vi "ShutdownCameraAndNIUSB.vi"(11 "Cluster":T3) -> ()   [LabVIEW 2024]
uses:
  <vilib>/vision/driver/NI_Vision_Acquisition_Software.lvlib
  <vilib>/userDefined/High Color/IMAQdx.ctl
  <vilib>/vision/Image Controls.llb/IMAQ Image.ctl
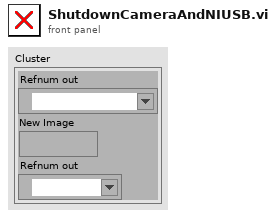
[diagram p1: front panel]
types:
  T1 = typedef "IMAQdx.ctl" = refnum<k21>
  T2 = typedef "IMAQ Image.ctl" = refnum<image>
  T3 = cluster{"Refnum out":T1, "New Image":T2, "Refnum out":refnum<k21>}
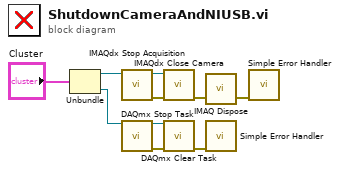
[diagram p0: block diagram]
diagram:
  n1 = Unbundle("Cluster") -> ("Refnum out"=w2:T1, "Refnum out"=w3:refnum<k21>)  [unwired: 1 out]
  n2 = call <vilib>:"IMAQdx Stop Acquisition.vi"("Session In"=w2) -> ("error out"=w5:errorcluster, "Session Out"=w9:T1)  [unwired: 9 in]
  n3 = call <vilib>:"DAQmx Stop Task.vi"("task/channels in"=w3) -> ("task out"=w8:refnum<k21>, "error out"=w6:errorcluster)  [unwired: 13 in]
  n4 = call <vilib>:"IMAQdx Close Camera.vi"("error in"=w5, "Session In"=w9) -> ("error out"=w4:errorcluster)  [unwired: 9 in]
  n5 = call <vilib>:"DAQmx Clear Task.vi"("task in"=w8, "error in"=w6) -> ("error out"=w7:errorcluster)  [unwired: 13 in]
  n6 = call "IMAQ Dispose"("error in (no error)"=w4) -> ("error out"=w10:errorcluster)  [unwired: 5 in]
  n7 = call <vilib>:"Simple Error Handler.vi"("error in (no error)"=w7) -> ()  [unwired: 4 in, 5 out]
  n8 = call <vilib>:"Simple Error Handler.vi"("error in (no error)"=w10) -> ()  [unwired: 4 in, 5 out]
